vi "SetBGColor.vi"(8 "error in":errorcluster, 10 "InitCluster_IN":T1, 11 "Background Color":u32(colorbox)) -> (0 "error out":errorcluster, 2 "InitCluster_OUT":T1)   [LabVIEW 2019]
uses:
  InitCluster.ctl
  CharacterCluster.ctl
  <vilib>/picture/picture.llb/imagedata.ctl
  ShotInitCluster.ctl
  <vilib>/Utility/miscctls.llb/LVPositionTypeDef.ctl
  <vilib>/Utility/miscctls.llb/LVBoundsTypeDef.ctl
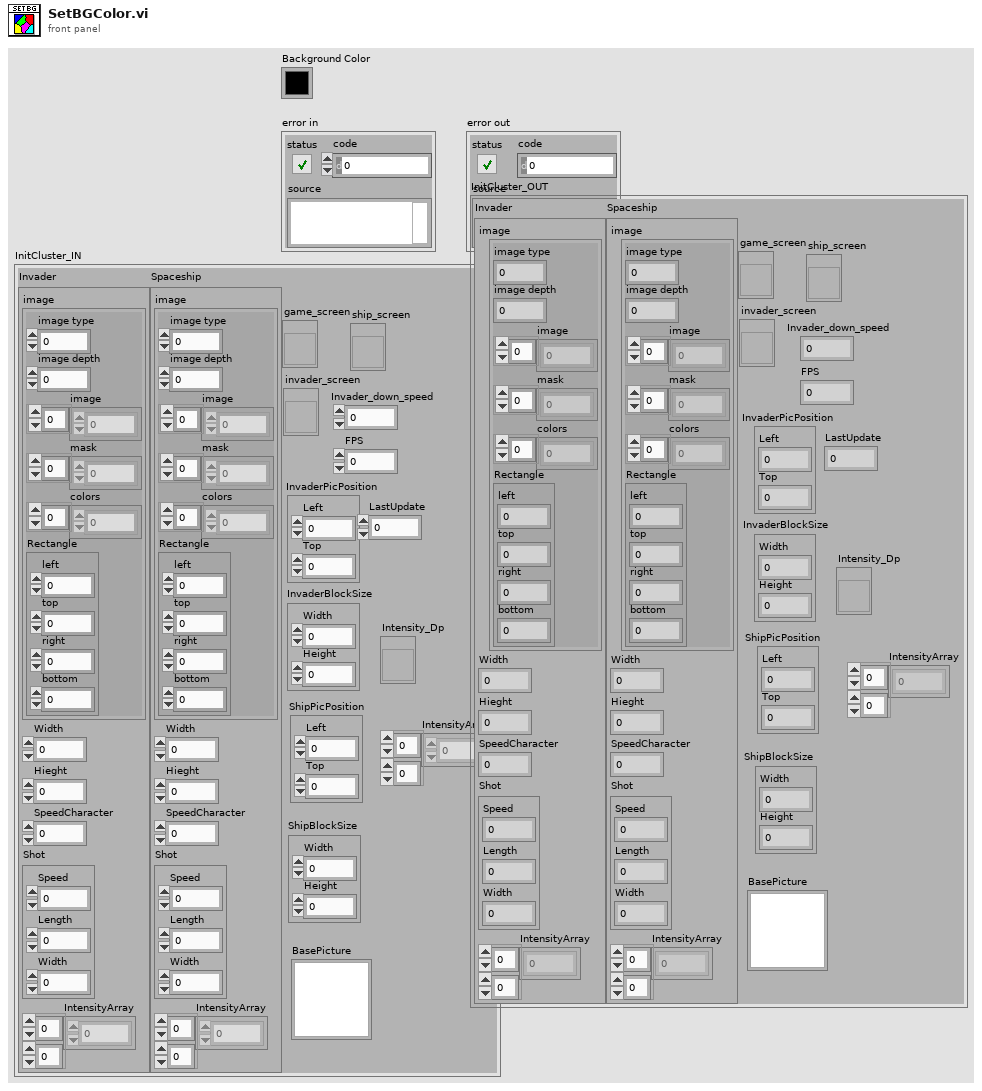
[diagram p1: front panel]
types:
  T1 = typedef "InitCluster.ctl" = cluster{"Invader":T2, "Spaceship":T2, "game_screen":refnum<vi>, "BasePicture":picture, "invader_screen":refnum<vi>, "InvaderPicPosition":T5, "Invader_down_speed":i16, "FPS":u16, "InvaderBlockSize":T6, "ship_screen":refnum<vi>, "ShipBlockSize":T6, "ShipPicPosition":T5, "LastUpdate":u32, "Intensity_Dp":refnum<vi>, "IntensityArray":u8[][]}
  T2 = typedef "CharacterCluster.ctl" = cluster{"image":T3, "Width":u32, "Hieght":u32, "SpeedCharacter":u32, "Shot":T4, "IntensityArray":u8[][]}
  T3 = typedef "imagedata.ctl" = cluster{"image type":i32, "image depth":i32, "image":u8[], "mask":u8[], "colors":u32[], "Rectangle":cluster{"left":i16, "top":i16, "right":i16, "bottom":i16}}
  T4 = typedef "ShotInitCluster.ctl" = cluster{"Speed":u32, "Length":u32, "Width":u32}
  T5 = typedef "LVPositionTypeDef.ctl" = cluster{"Left":i32, "Top":i32}
  T6 = typedef "LVBoundsTypeDef.ctl" = cluster{"Width":u32, "Height":u32}
  T7 = cluster{"left":i16, "top":i16, "right":i16, "bottom":i16}
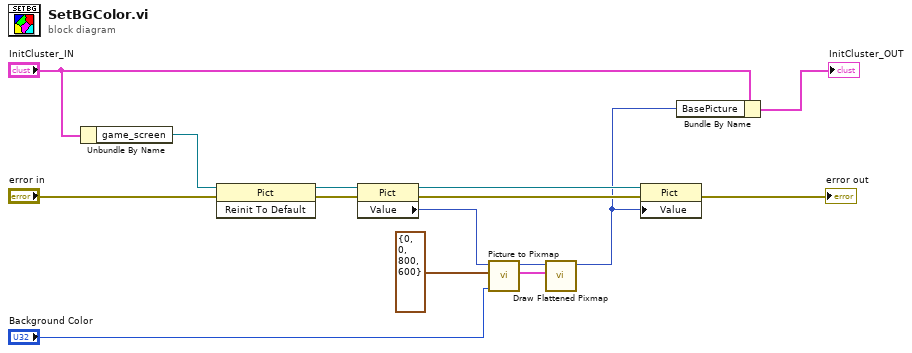
[diagram p0: block diagram]
diagram:
  n1 = Unbundle By Name("InitCluster_IN") -> ("game_screen"=w7:refnum<vi>)
  n2 = invoke class="Pict" method="Reinit To Default"(reference=w7, error in="error in") -> (reference out=w5:refnum<vi>, error out=w4:errorcluster)  [unwired: 1 in, 1 out]
  n3 = property class="Pict"(reference=w5, error in=w4) -> (reference out=w14:refnum<vi>, error out=w13:errorcluster, "Value"=w12:picture)
  n4 = call <vilib>:"Picture to Pixmap.vi"("Background Color"="Background Color", "rect"=T7 {"left"=0, "top"=0, "right"=800, "bottom"=600}, "picture"=w12) -> ("image data"=w10:T3, "new picture"=w9:picture)  [unwired: 7 in]
  n5 = call <vilib>:"Draw Flattened Pixmap.vi"("image data"=w10, "picture"=w9) -> ("new picture"=w3:picture)  [unwired: 7 in]
  n6 = property class="Pict"(reference=w14, error in=w13, "Value"=w3) -> (error out=→"error out":errorcluster)  [unwired: 1 out]
  n7 = Bundle By Name(cluster="InitCluster_IN", "BasePicture"=w3) -> (→"InitCluster_OUT":T1)
